vi "MoAgSy_Host_GPG_keyring.vi"(0 "Host_Reference":refnum<class "HGF_Reference.lvclass">, 2 "key":string, 5 "error in (no error)":errorcluster, 6 "timeout in ms (-1)":i32=-1, 8 "task":T1(ring)) -> (14 "dup Host_Reference":refnum<class "HGF_Reference.lvclass">, 19 "error out":errorcluster)   [LabVIEW 2009, in "MoAgSy.lvlib" / "MoAgSy_Host.lvclass"]
uses:
  MoAgSy_Host.lvclass
  HGF_BaseClasses/HGF_Reference/HGF_Reference.lvclass
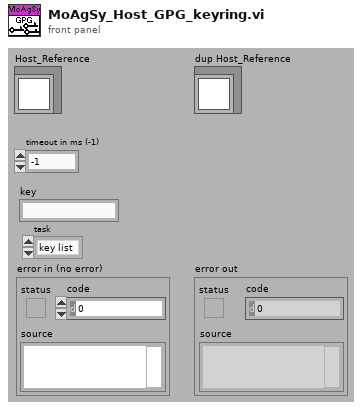
[diagram p1: front panel]
types:
  T1 = enum16{"key list", "pub key", "delete key", "add key", "local sign key"}
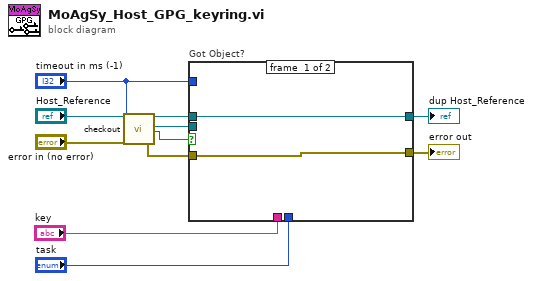
[diagram p0: block diagram]
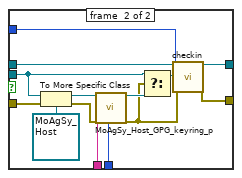
[diagram p2: hidden frame]
diagram:
  n1 = call "checkout.vi"("HGF_Reference"="Host_Reference", "timeout in ms (-1)"="timeout in ms (-1)", "error in (no error)"="error in (no error)") -> ("dup HGF_Reference"=w6:refnum<class "HGF_Reference.lvclass">, "Object"=w9:refnum<class>, "got object?"=w7:bool, "error out"=w10:errorcluster)  [unwired: 13 out]
  n2 = case "Got Object?" shown="True" w7 {
    tunnel: w10 -> [w12 w27]
    tunnel: w9 -> [_ w21]
    tunnel: w6 -> [w13 w25]
    tunnel: [w13 w24] -> w5
    tunnel: "timeout in ms (-1)" -> [_ w23]
    tunnel: [w12 w22] -> w3
    tunnel: "key" -> [_ w15]
    tunnel: "task" -> [_ w14]
    frame #0 {
    }
    frame #1 {
      n3 = To More Specific Class(target class=refnum<class "MoAgSy_Host.lvclass"> refnum ("MoAgSy.lvlib:MoAgSy_Host.lvclass"), reference=w21, error in=w27) -> (specific class reference=w19:refnum<class "MoAgSy_Host.lvclass">, error out=w16:errorcluster)
      n4 = call "MoAgSy_Host_GPG_keyring_p.vi"("MoAgSy_Host"=w19, "key"=w15, "error in (no error)"=w16, "task"=w14) -> ("dup MoAgSy_Host"=w18:refnum<class "MoAgSy_Host.lvclass">, "error out"=w17:errorcluster)  [unwired: 12 in, 2 out]
      n5 = Select(t=w21, s=w17, f=w18) -> (s? t:f=w20:refnum<class>)
      n6 = call "checkin.vi"("HGF_Reference"=w25, "Object"=w20, "timeout /ms (-1)"=w23, "error in (no error)"=w17) -> ("dup HGF_Reference"=w24:refnum<class "HGF_Reference.lvclass">, "error out"=w22:errorcluster)  [unwired: 14 out]
    }
  }
  "dup Host_Reference" <- w5
  "error out" <- w3
